vi "unary_client.vi"() -> ()   [LabVIEW 2019]
uses:
  Generated_client/RPC Messages/Request.ctl
  Generated_client/RPC Messages/Request_request_oneof/Request_request_oneof.lvclass
  Generated_client/RPC Messages/Request_request_oneof/Request_request_oneof.lvclass/Request_request_oneof.ctl
  Generated_client/RPC Messages/Response_response_oneof/Response_response_oneof.lvclass/Response_response_oneof.ctl
  Generated_client/Generated_client.lvlib
  Generated_client/RPC Messages/Response_response_oneof/Response_response_oneof.lvclass
panel:
  out "resp_id":i32
  out "result":string
  out "new_age":i32
  in  "age":i32
  in  "message":string
  in  "req_id":i32
  in  "req_oneof":enum16{"message", "req_id"}(ring)
  out "error out":errorcluster
  in  "error in":errorcluster
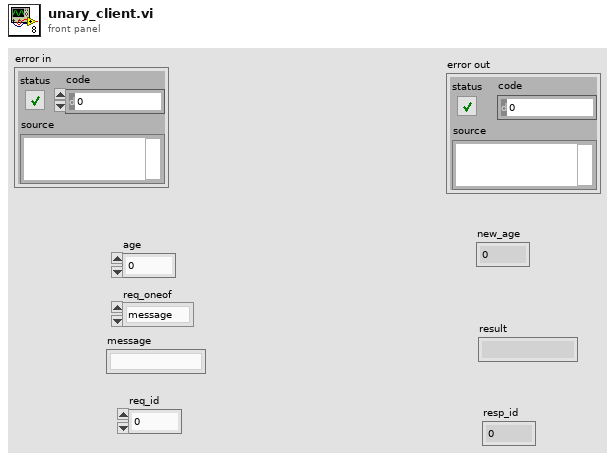
[diagram p1: front panel]
types:
  T1 = typedef "Generated_client.lvlib/Request.ctl" = cluster{"age":i32, "Request_request_oneof":refnum<class "Request_request_oneof.lvclass">}
  T2 = typedef "grpc-lvsupport-release.lvlib/grpcId.ctl" = u64
  T3 = typedef "Generated_client.lvlib/Response.ctl" = cluster{"new_age":i32, "Response_response_oneof":refnum<class "Response_response_oneof.lvclass">}
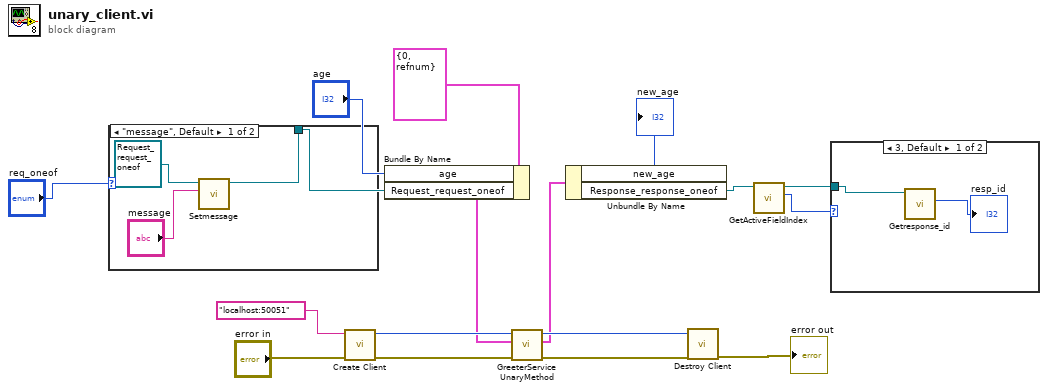
[diagram p0: block diagram]
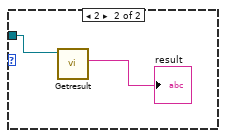
[diagram p2: hidden frame]
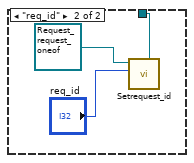
[diagram p3: hidden frame]
diagram:
  n1 = case shown="\"message\", Default" "req_oneof" {
    tunnel: [w18 w21] -> w8
    frame "message", Default {
      n2 = call "Setmessage.vi"("Set_Val"="message", "OneOfTemplate in"=refnum<class "Request_request_oneof.lvclass"> refnum) -> ("OneOfTemplate out"=w18:refnum<class "Request_request_oneof.lvclass">)  [unwired: 8 in, 1 out]
    }
    frame "req_id" {
      n3 = call "Setrequest_id.vi"("Set_Val"="req_id", "OneOfTemplate in"=refnum<class "Request_request_oneof.lvclass"> refnum) -> ("OneOfTemplate out"=w21:refnum<class "Request_request_oneof.lvclass">)  [unwired: 8 in, 1 out]
    }
  }
  n4 = call "Create Client.vi"("error in"="error in", "address"="localhost:50051") -> ("error out"=w14:errorcluster, "gRPC ID Out"=w17:T2)  [unwired: 8 in]
  n5 = Bundle By Name(cluster=T1 {"age"=0, "Request_request_oneof"=refnum} ("Request"), "age"="age", "Request_request_oneof"=w8) -> (w6:T1)
  n6 = call "GreeterService UnaryMethod.vi"("error in"=w14, "Request Data"=w6, "gRPC ID"=w17) -> ("error out"=w13:errorcluster, "Response Data"=w5:T3, "gRPC ID out"=w16:T2)  [unwired: 6 in]
  n7 = Unbundle By Name(w5) -> ("new_age"=→"new_age":i32, "Response_response_oneof"=w3:refnum<class "Response_response_oneof.lvclass">)
  n8 = call "Destroy Client.vi"("error in"=w13, "gRPC ID"=w16) -> ("error out"=→"error out":errorcluster)  [unwired: 9 in]
  n9 = call "GetActiveFieldIndex.vi"("OneOfTemplate in"=w3) -> ("Active Field Index"=w1:i32, "OneOfTemplate out"=w2:refnum<class "Response_response_oneof.lvclass">)  [unwired: 8 in, 1 out]
  n10 = case shown="3, Default" w1 {
    tunnel: w2 -> [w25 w26]
    frame 3, Default {
      n11 = call "Getresponse_id.vi"("OneOfTemplate in"=w25) -> ("Get_Val"=→"resp_id":i32)  [unwired: 8 in, 2 out]
    }
    frame 2 {
      n12 = call "Getresult.vi"("OneOfTemplate in"=w26) -> ("Get_Val"=→"result":string)  [unwired: 8 in, 2 out]
    }
  }
